vi "模拟输入_RTD或热敏电阻_连续.vi"() -> ()   [LabVIEW 2013]
doc: "This example demonstrates how to acquire a continuous data."
uses:
  <userlib>/ArtDAQ/_SubVI/ArtDAQ_CfgSampClkTiming.vi
  <userlib>/ArtDAQ/_SubVI/ArtDAQ_CreateAIRTDChan.vi
  <userlib>/ArtDAQ/_SubVI/ArtDAQ_CreateAIThrmstrChanIex.vi
  <userlib>/ArtDAQ/_SubVI/ArtDAQ_Read Analog DBL NChan NSamp.vi
panel:
  in  "电流激励源":i32(ring)=10167 items=["内部"=10200, "外部"=10167, "无"=10230]
  in  "电阻配置":i32(ring)=4 items=["2-线"=2, "3-线"=3, "4-线"=4]
  in  "最小值(°C)":dbl format="%0.2f"
  in  "最大值(°C)":dbl=100.0 format="%0.2f"
  in  "电流激励值":dbl=0.004 format="%0.3f"
  in  "选项卡控件":enum32{"RTD", "Thermistor"}(tab)
  in  "RTD参数":cluster{"0摄氏度时传感器的电阻":dbl, "RTD类型":i32}={"0摄氏度时传感器的电阻"=100.0, "RTD类型"=12481} {"RTD类型" items=["Pt3750"=12481, "Pt3851"=10071, "Pt3911"=12482, "Pt3916"=10069, "Pt3920"=10053, "Pt3928"=12483, "自定义"=10137]; "0摄氏度时传感器的电阻" format="%1_5g"}
  in  "热敏电阻参数":cluster{"A":dbl, "B":dbl, "C":dbl}={"A"=0.001295361, "B"=0.0002343159, "C"=1.018703e-07} {"C" format="%^0.5e"; "B" format="%^0.5e"; "A" format="%^0.5e"}
  in  "停止":bool
  out "Waveform":dbl[][](graph)
  in  "采样频率":dbl=10000.0 format="%#_13g"
  in  "每通道采样点数":i32=1000
  in  "物理通道":string(combo)="Dev1/ai0"
  out "错误":errorcluster
  # "通道属性"
  # "定时"
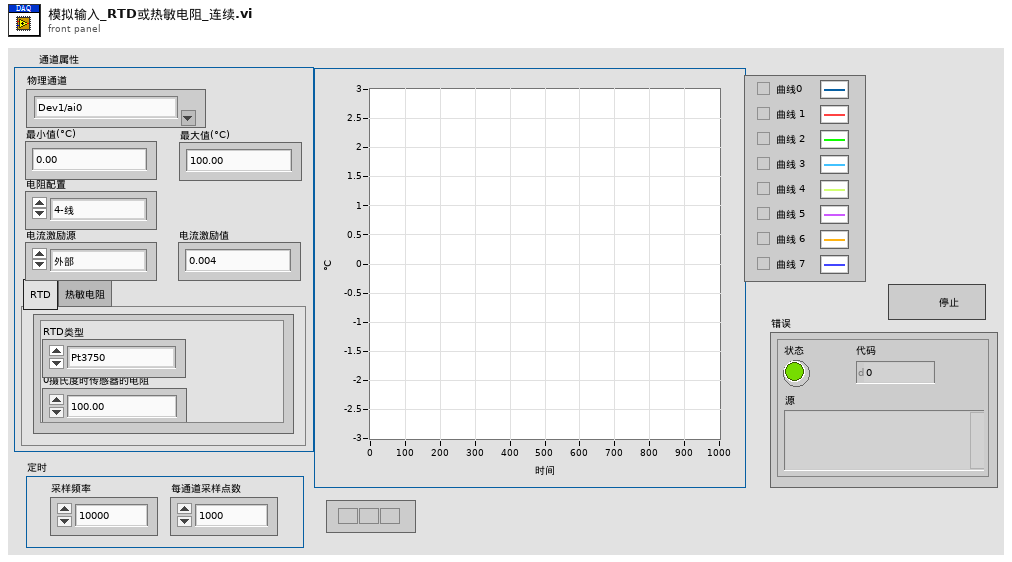
[diagram p1: front panel]
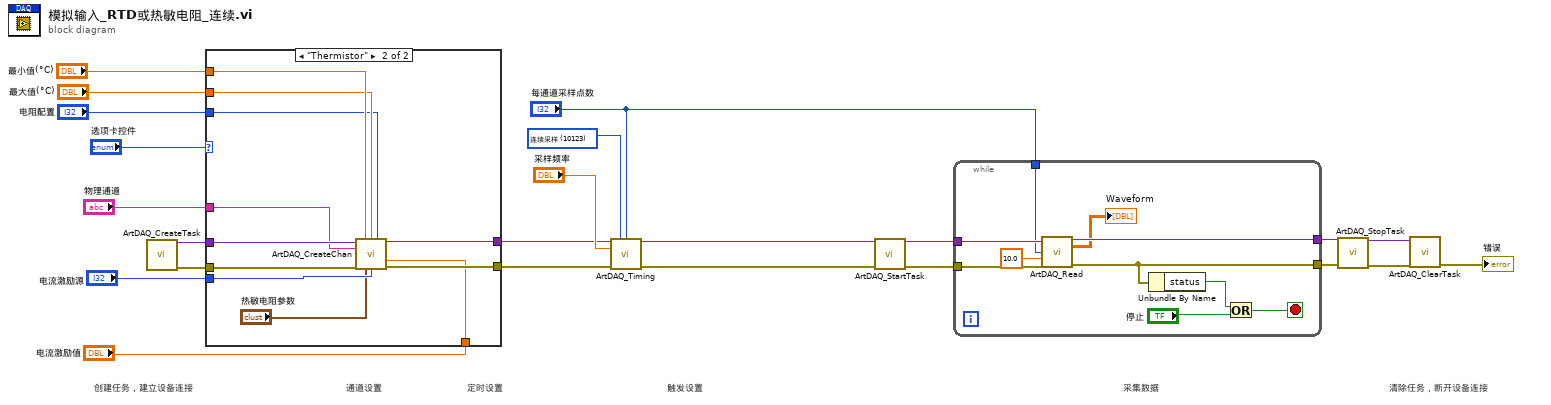
[diagram p0: block diagram]
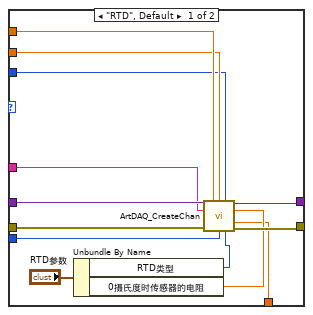
[diagram p2: hidden frame]
diagram:
  w9 = 10123 items=["有限点采样"=10178, "连续采样"=10123] ("SampleMode")
  # "清除任务，断开设备连接"
  # "采集数据"
  # "触发设置"
  # "定时设置"
  # "通道设置"
  # "创建任务，建立设备连接"
  n1 = call <userlib>:"ArtDAQ_CreateTask.vi"() -> ("任务句柄"=w16:variant, "错误输出"=w23:errorcluster)  [unwired: 14 in]
  n2 = case shown="\"Thermistor\"" "选项卡控件" {
    tunnel: w23 -> [w34 w47]
    tunnel: [w33 w46] -> w22
    tunnel: w16 -> [w36 w45]
    tunnel: "物理通道" -> [w26 w44]
    tunnel: [w35 w43] -> w10
    tunnel: "最小值(°C)" -> [w29 w42]
    tunnel: "最大值(°C)" -> [w28 w41]
    tunnel: "电阻配置" -> [w27 w40]
    tunnel: "电流激励源" -> [w25 w39]
    tunnel: "电流激励值" -> [w24 w38]
    frame "RTD", Default {
      n3 = Unbundle By Name("RTD参数") -> ("RTD类型"=w31:i32, "0摄氏度时传感器的电阻"=w30:dbl)
      n4 = call-poly <userlib>:"ArtDAQ_CreateChan.vi"("任务句柄"=w36, "最小值"=w29, "最大值"=w28, "电阻配置"=w27, "物理通道"=w26, "r0"=w30, "电流激励值"=w24, "错误输入"=w34, "电流激励源"=w25, "RTD 类型"=w31) -> ("任务句柄"=w35:variant, "错误输出"=w33:errorcluster)  [unwired: 4 in]
    }
    frame "Thermistor" {
      n5 = call-poly <userlib>:"ArtDAQ_CreateChan.vi"("任务句柄"=w45, "最小值"=w42, "最大值"=w41, "电阻配置"=w40, "物理通道"=w44, "电流激励值"=w38, "错误输入"=w47, "热敏电阻特性"="热敏电阻参数", "电流激励源"=w39) -> ("任务句柄"=w43:variant, "错误输出"=w46:errorcluster)  [unwired: 5 in]
    }
  }
  n6 = call-poly <userlib>:"ArtDAQ_Timing.vi"("任务句柄"=w10, "采样模式"=w9, "每通道采样数"="每通道采样点数", "采样率"="采样频率", "错误输入"=w22) -> ("任务句柄"=w8:variant, "错误输出"=w7:errorcluster)  [unwired: 9 in]
  n7 = call <userlib>:"ArtDAQ_StartTask.vi"("任务句柄"=w8, "错误输入"=w7) -> ("任务句柄"=w19:variant, "错误输出"=w18:errorcluster)  [unwired: 12 in]
  n8 = while {
    tunnel: w19 -> [w57]
    tunnel: w18 -> [w56]
    tunnel: "每通道采样点数" -> [w55]
    tunnel: [w53] -> w15
    tunnel: [w52] -> w14
    stop <- w50 stop-if-true
    n9 = call-poly <userlib>:"ArtDAQ_Read.vi"("任务句柄"=w57, "每通道采样数"=w55, "超时s"=10.0 ("Timeout"), "错误输入"=w56) -> ("任务句柄"=w53:variant, "数据"=→"Waveform":dbl[][], "错误输出"=w52:errorcluster)  [unwired: 8 in, 1 out]
    n10 = Unbundle By Name(w52) -> ("status"=w51:bool)
    n11 = Or(x=w51, y="停止") -> (x .or. y?=w50:bool)
  }
  n12 = call <userlib>:"ArtDAQ_StopTask.vi"("任务句柄"=w15, "错误输入"=w14) -> ("任务句柄"=w13:variant, "错误输出"=w12:errorcluster)  [unwired: 12 in]
  n13 = call <userlib>:"ArtDAQ_ClearTask.vi"("任务句柄"=w13, "错误输入"=w12) -> ("错误输出"=→"错误":errorcluster)  [unwired: 13 in]
